vi "resonance scan engine 4 channel fixed pixel clock acquisition (Host).vi"() -> ()   [LabVIEW 2012]
uses:
  <vilib>/rvi/interface/nirviMethod/nirviMethod.xnode
  <vilib>/rvi/interface/nirviCloseFPGA/nirviCloseFPGA.xnode
  4 ch resonance scanner acquisition fixed pixel clock Folder/D/gitrepo/140812_ssdev_repo/FPGA/current bitfiles/4chresonancescan_PXIe-7962R_newLindsaymod4ch_VaUfink3TSc.lvbitx
  <vilib>/FPGAPlugInAG/PXIe-7962R/niLvFpga_AcknowledgeIrq_PXIe-7962R.vi
  <vilib>/rvi/interface/nirviMethod/StockFPGA_InlinedMethodWaitForSingleIRQ.vi
  <vilib>/FPGAPlugInAG/PXIe-7962R/niLvFpga_WaitOnIrq_PXIe-7962R.vi
  <vilib>/FPGAPlugInAG/PXIe-7962R/niLvFpga_ReadFifo_PXIe-7962R.vi
  <vilib>/rvi/errors/niLvFpgaMergeErrorWithErrorCode.vi
  <vilib>/FPGAPlugInAG/PXIe-7962R/niLvFpga_Close_PXIe-7962R.vi
panel:
  in  "x resonant zoom voltage":dbl
  in  "y-voltage":dbl=2.0
  out "max":u32
  out "x-y":u32
  out "error out":errorcluster
  in  "stop":bool
  in  "lines (2pi) per frame":i32=100
  in  "Start Delay (Ticks)":i16
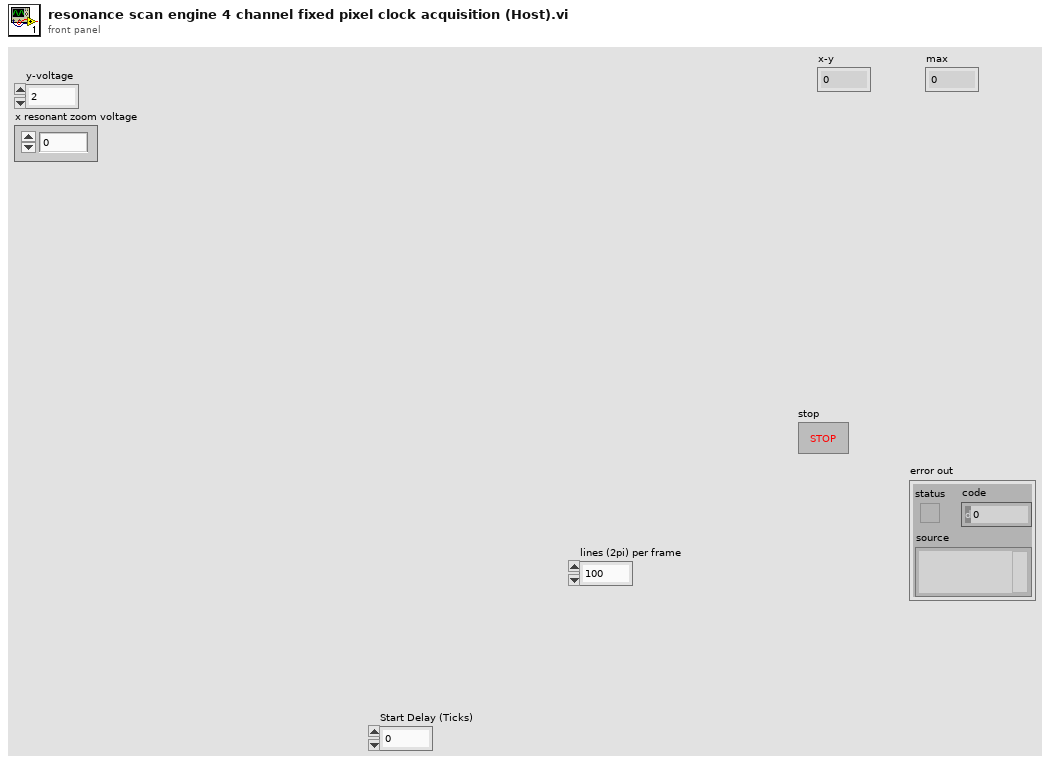
[diagram p1: front panel]
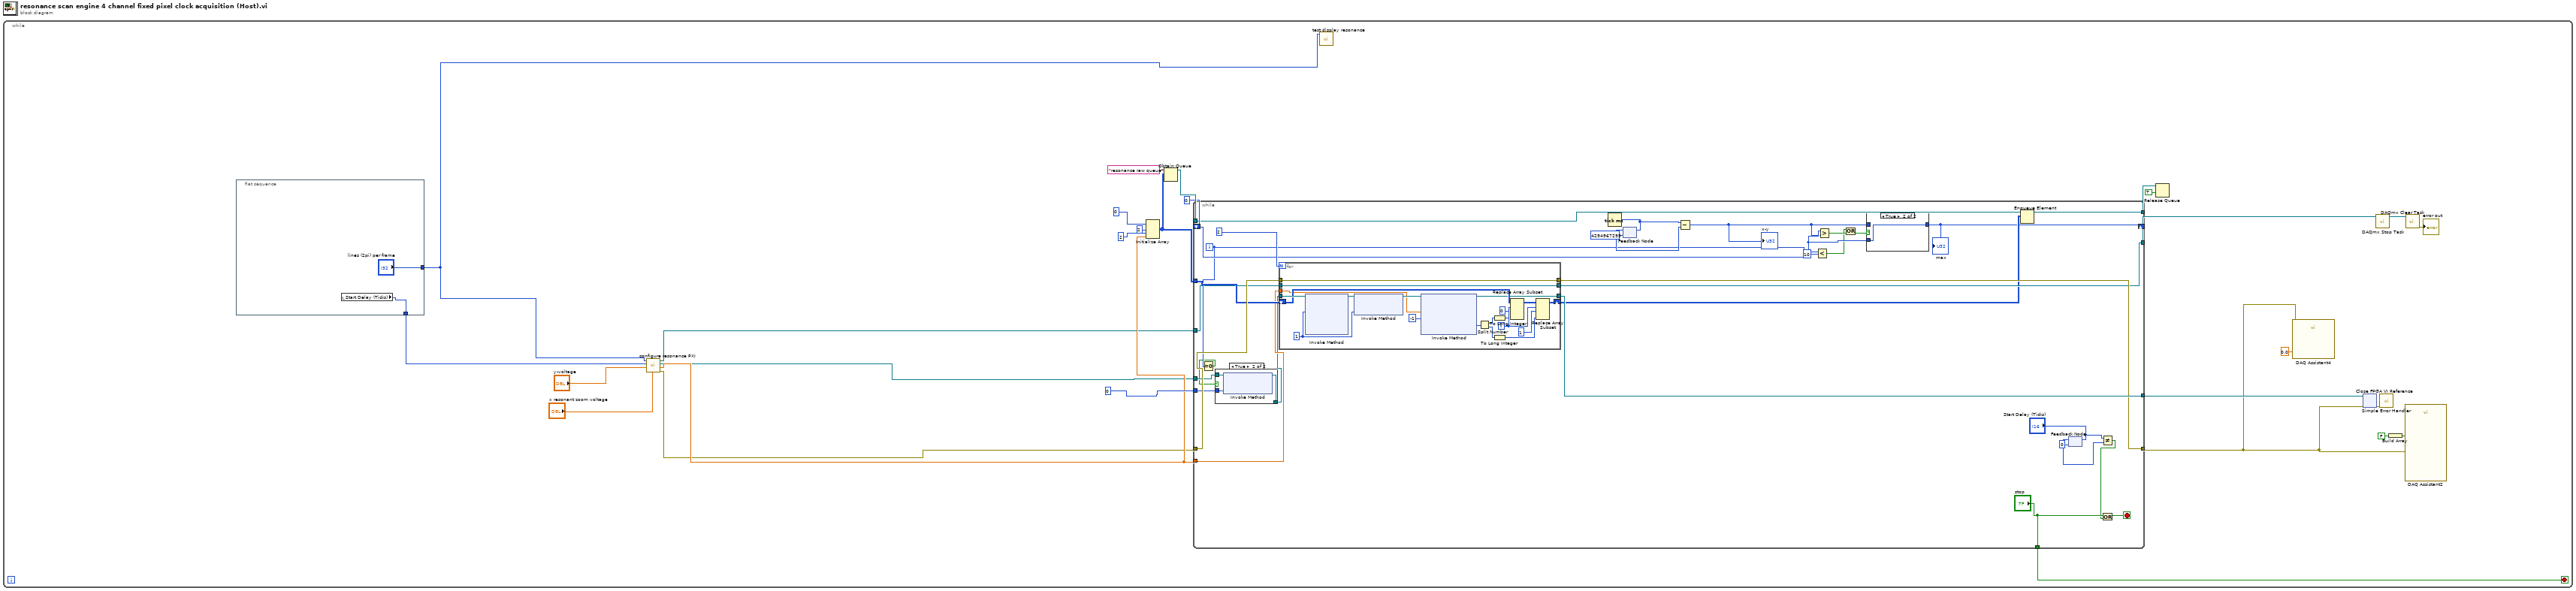
[diagram p0: block diagram]
diagram:
  n1 = while {
    stop <- w9 stop-if-true
    n2 = flat-sequence {
      tunnel: ["lines (2pi) per frame"] -> w5
      tunnel: [w29] -> w4
      frame #0 {
        n3 = local read "Start Delay (Ticks)"() -> (w29:i16)
      }
    }
    n4 = call "configure resonance PXI.vi"("x resonant zoom voltage"="x resonant zoom voltage", "y-voltage"="y-voltage", "Start Delay (Ticks)"=w4, "lines (2pi) per frame"=w5) -> ("error out"=w2:errorcluster, "pixels per frame"=w8:dbl, "FPGA VI Reference Out"=w6:refnum<k20>, "AO task out"=w7:refnum<k21>)  [unwired: 3 in, 1 out]
    n5 = Initialize Array(0, 2 ("dimension size"), 2 ("dimension size"), w8) -> (w18:i32[][][])
    n6 = Obtain Queue(name (unnamed)="resonance raw queue", element data type=w18) -> (queue out=w16:refnum<queue>)  [unwired: 3 in, 2 out]
    n7 = while {
      tunnel: w2 -> [w62]
      tunnel: [w61] -> w25
      tunnel: [w60] -> w12
      tunnel: [w59] -> w23
      tunnel: w6 -> [w40]
      tunnel: w7 -> [w37]
      tunnel: w18 -> [w57]
      tunnel: w8 -> [w56]
      tunnel: w16 -> [w54]
      tunnel: [w53] -> w15
      shift-right: [w47] -> _
      shift-left: u32 0 -> [w49]
      tunnel: 0 ("IRQ Number(s)") -> [w41]
      tunnel: ["stop"] -> w9
      i -> [w42]
      stop <- w33 stop-if-true
      n8 = Equal To 0?(x=w42) -> (x = 0?=w38:bool)
      n9 = case shown="True" w38 {
        tunnel: w41 -> [_ w66]
        tunnel: w40 -> [w63 w65]
        tunnel: [w63 w64] -> w39
        frame False {
        }
        frame True {
          n10 = xnode "Invoke Method"("FPGA VI Reference In"=w65, "IRQ Number(s)"=w66) -> ("FPGA VI Reference Out"=w64:refnum<k20>)  [unwired: 1 in, 1 out]
        }
      }
      n11 = for {
        N: 2 -> [_]
        tunnel: [w82] -> w61
        tunnel: [w88] -> w60
        tunnel: [w71] -> w59
        tunnel: w62 -> [w88]
        tunnel: w37 -> [w71]
        tunnel: w56 -> [w79]
        tunnel: w39 -> [w87]
        shift-right: [w80] -> w55
        shift-left: w57 -> [w84]
        i -> [w81]
        w70 = 1 ("IRQ Number(s)")
        n12 = xnode "Invoke Method"("FPGA VI Reference In"=w87, "IRQ Number(s)"=w70) -> ("FPGA VI Reference Out"=w69:refnum<k20>)  [unwired: 2 in, 3 out]
        n13 = xnode "Invoke Method"("FPGA VI Reference In"=w69, "IRQ Number(s)"=w70) -> ("FPGA VI Reference Out"=w86:refnum<k20>)  [unwired: 1 in, 1 out]
        n14 = xnode "Invoke Method"("FPGA VI Reference In"=w86, "Number of Elements"=w79, "Timeout (ms)"=-1) -> ("FPGA VI Reference Out"=w82:refnum<k20>, "Data"=w85:u64[])  [unwired: 1 in, 2 out]
        n15 = Split Number(x=w85) -> (hi(x)=w78:u32[], lo(x)=w77:u32[])
        n16 = To Long Integer(number=w78) -> (32bit integer=w73:i32[])
        n17 = To Long Integer(number=w77) -> (32bit integer=w72:i32[])
        n18 = Replace Array Subset(array=w84, new element=w73, index (dim 0)=w81, index (dim 1)=0 ("disabled index (row)")) -> (w76:i32[][][])  [unwired: 1 in]
        n19 = Replace Array Subset(array=w76, new element=w72, index (dim 0)=w81, index (dim 1)=1 ("disabled index (row)")) -> (w80:i32[][][])  [unwired: 1 in]
      }
      n20 = Tick Count (ms)() -> (millisecond timer value=w52:u32)
      n21 = feedback-in #1(w52) -> ()
      n22 = feedback #1(u32 4294967295 ("millisecond timer value")) -> (w51:u32)
      n23 = Subtract(x=w52, y=w51) -> (x-y=w48:u32)
      "x-y" <- w48
      n24 = Less?(x=w42, y=10) -> (x < y?=w44:bool)
      n25 = Greater?(x=w49, y=w48) -> (0:w50:bool)
      n26 = Or(x=w44, y=w50) -> (x .or. y?=w45:bool)
      n27 = case shown="True" w45 {
        tunnel: w49 -> [_ w68]
        tunnel: w48 -> [w67 _]
        tunnel: [w67 w68] -> w47
        frame False {
        }
        frame True {
        }
      }
      "max" <- w47
      n28 = Enqueue Element(queue=w54, element=w55) -> (queue out=w53:refnum<queue>)  [unwired: 2 in, 2 out]
      n29 = feedback-in #2("Start Delay (Ticks)") -> ()
      n30 = feedback #2(i16 0 ("Start Delay (Ticks)")) -> (w34:i16)
      n31 = Not Equal?(x="Start Delay (Ticks)", y=w34) -> (x != y?=w32:bool)
      n32 = Or(x="stop", y=w32) -> (x .or. y?=w33:bool)
    }
    n33 = call "test display resonance.vi"("lines (2pi) per frame"=w5) -> ()  [unwired: 11 in]
    n34 = Release Queue(queue=w15, force destroy? (F)=TRUE) -> ()  [unwired: 1 in, 3 out]
    n35 = call "DAQ Assistant4"("data"=0.0, "error in"=w12) -> ()  [unwired: 16 in, 2 out]
    n36 = xnode "Close FPGA VI Reference"("FPGA VI Reference In"=w25, "error in"=w12) -> ("error out"=w26:errorcluster)
    n37 = call <vilib>:"DAQmx Stop Task.vi"("task/channels in"=w23) -> ("task out"=w22:refnum<k21>)  [unwired: 13 in, 1 out]
    n38 = call <vilib>:"Simple Error Handler.vi"("error in (no error)"=w26) -> ()  [unwired: 1 in, 8 out]
    n39 = Build Array(FALSE) -> (w28:bool[])
    n40 = call "DAQ Assistant2"("data"=w28, "error in"=w12) -> ()  [unwired: 16 in, 2 out]
    n41 = call <vilib>:"DAQmx Clear Task.vi"("task in"=w22) -> ("error out"=→"error out":errorcluster)  [unwired: 14 in]
  }
